vi "mapStringToNumber.vi"(11 "Array":string[](array[string])) -> (3 "value":i32[](array[numeric]))   [LabVIEW 2026]
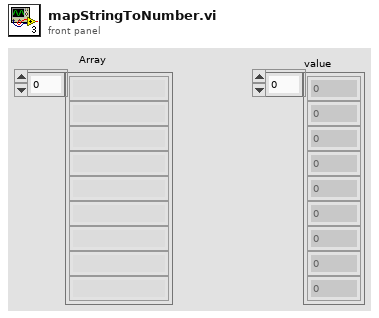
[diagram p1: front panel]
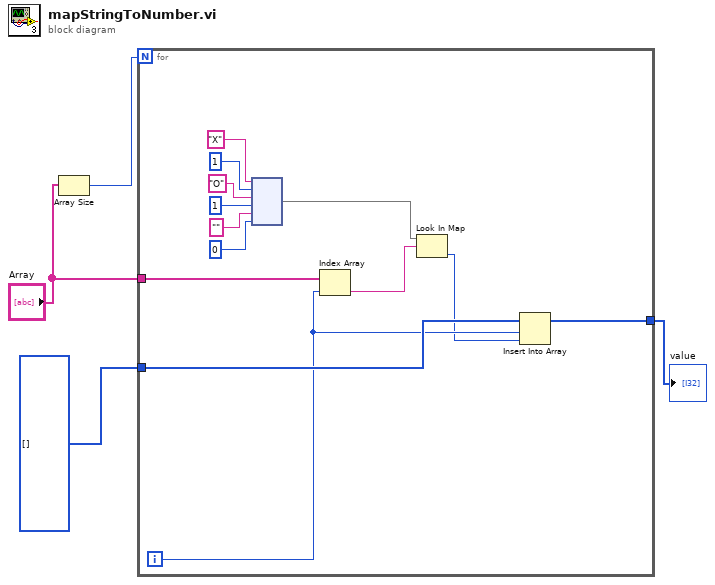
[diagram p0: block diagram]
diagram:
  n1 = Array Size(array="Array") -> (size(s)=w4:i32)
  n2 = for {
    N: w4 -> [_]
    tunnel: "Array" -> [w10]
    tunnel: i32[] [] -> [w8]
    tunnel: [w5] -> w1
    i -> [w7]
    n3 = node("X" ("key"), 1 ("value"), "O" ("key"), 1 ("value"), "" ("key"), 0 ("value")) -> (w17:map{string, i32})
    n4 = Index Array(array=w10, index=w7) -> (element=w9:string)
    n5 = Look In Map(map=w17, key=w9) -> (value=w6:i32)  [unwired: 1 in, 1 out]
    n6 = Insert Into Array(array=w8, index=w7, new element=w6) -> (w5:i32[])
  }
  "value" <- w1
